vi "CheckValues.vi"(8 "error in (no error)":errorcluster, 11 "NHRDCPower in":refnum<class "NHRDCPower.lvclass">) -> (0 "error out":errorcluster, 3 "NHRDCPower out":refnum<class "NHRDCPower.lvclass">)   [LabVIEW 2018, in "AcPwrPlugins.lvlib" / "NHRDCPower.lvclass"]
uses:
  NHRDCPower.lvclass
  <vilib>/Utility/error.llb/Error Cluster From Error Code.vi
  <vilib>/ErrorRing/Error Ring.xnode
  <instrlib>/NHRDCPowerModule/NHRDCPowerModule/NHRDCPowerModule.lvlib
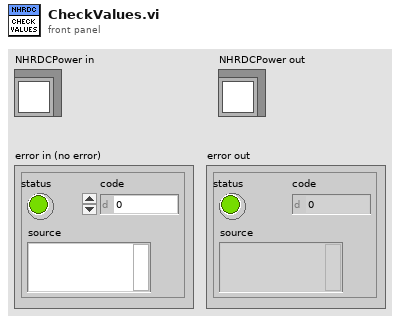
[diagram p1: front panel]
types:
  T1 = typedef "AcPwrPlugins.lvlib/NHRDCPower.lvclass/Device(s)Settings.ctl" = cluster{"Handle":string, "Name":string, "Phase Select":i32, "id query (Yes)":bool, "reset device (Yes)":bool, "Connected":bool, "Voltage Range (V)":dbl[], "Timing":cluster{"TimingOn":enum16{""}, "Hours":u32, "Minutes":u32, "Seconds":dbl, "CutoffVoltage":dbl}, "Simulate Instrument(T)":bool, "SlewRate":cluster{"Set Voltage Rate V/S":sgl, "Set Current Rate A/S":sgl, "Set Resistance Rate R/S":sgl, "Set Power Rate W/S":sgl}, "OutputSettings":cluster{"operating state (Off)":i32, "Voltage (V)":sgl, "Current (A)":sgl, "Resistance (Ohms)":sgl, "Power (W)":sgl, "Enable Voltage":bool, "Enable Current":bool, "Enable Resistance":bool, "Enable Power":bool, "Aperture Time (s)":sgl}, "Initial Battery Detect Voltage (0)":dbl, "SafetySettings":cluster{"SetWatchDog":bool, "Voltage (V)":sgl, "Current (A)":sgl, "Power (W)":sgl, "Voltage Delay (s)":sgl, "Current Delay (s)":sgl, "Power Delay (s)":sgl}}[]
  T2 = cluster{"Set Voltage Rate V/S":sgl, "Set Current Rate A/S":sgl, "Set Resistance Rate R/S":sgl, "Set Power Rate W/S":sgl}
  T3 = cluster{"operating state (Off)":i32, "Voltage (V)":sgl, "Current (A)":sgl, "Resistance (Ohms)":sgl, "Power (W)":sgl, "Enable Voltage":bool, "Enable Current":bool, "Enable Resistance":bool, "Enable Power":bool, "Aperture Time (s)":sgl}
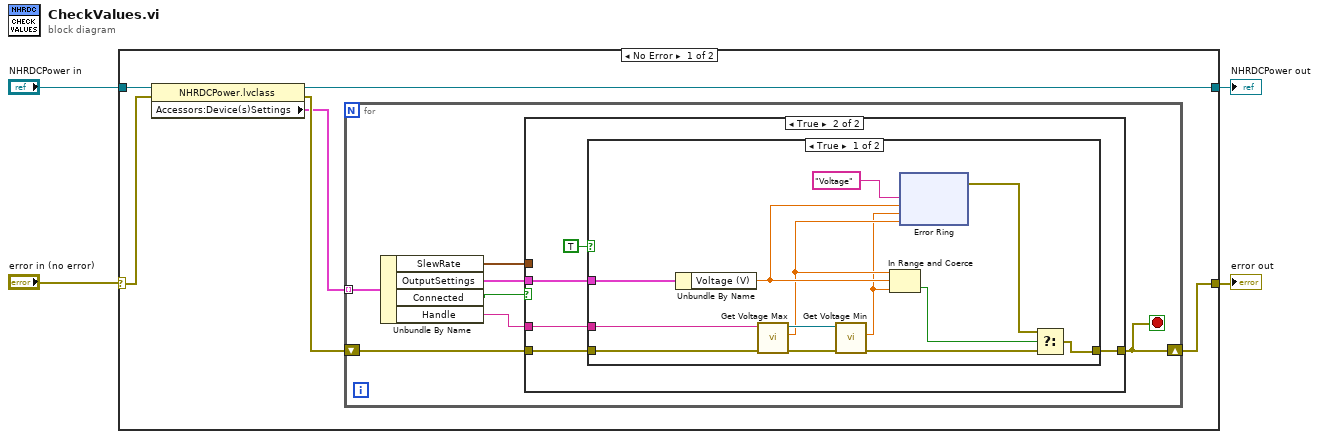
[diagram p0: block diagram]
diagram:
  n1 = case shown="No Error" "error in (no error)" {
    selector: "error in (no error)" -> [w9 w49]
    tunnel: [w8 w49] -> w1
    tunnel: [w10 w48] -> w3
    tunnel: "NHRDCPower in" -> [w6 w48]
    frame No Error {
      n2 = property class="NHRDCPower.lvclass"(reference=w6, error in=w9) -> (reference out=w10:refnum<class "NHRDCPower.lvclass">, error out=w7:errorcluster, "Accessors:Device(s)Settings"=w5:T1)
      n3 = for {
        tunnel: w5 -> [w17] mode=indexing
        shift-right: [w15] -> w8
        shift-left: w7 -> [w16]
        stop <- w15 stop-if-true
        n4 = Unbundle By Name(w17) -> ("SlewRate"=w11:T2, "OutputSettings"=w12:T3, "Connected"=w13:bool, "Handle"=w14:string)
        n5 = case shown="True" w13 {
          tunnel: w16 -> [w18 w23]
          tunnel: [w18 w20] -> w15
          tunnel: w14 -> [_ w22]
          tunnel: w12 -> [_ w21]
          tunnel: w11 -> [_ _]
          frame False {
          }
          frame True {
            n6 = case shown="True" TRUE {
              tunnel: w23 -> [w36 w47]
              tunnel: w22 -> [w35 _]
              tunnel: w21 -> [w32 _]
              tunnel: [w27 w47] -> w20
              frame True {
                n7 = Unbundle By Name(w32) -> ("Voltage (V)"=w31:sgl)
                n8 = call <instrlib>:"Get Voltage Max.vi"("error in (no error)"=w36, "instrument handle"=w35) -> ("error out"=w33:errorcluster, "maximum voltage"=w30:sgl, "instrument handle out"=w34:refnum<visa-resource-name>)  [unwired: 7 in]
                n9 = call <instrlib>:"Get Voltage Min.vi"("error in (no error)"=w33, "instrument handle"=w34) -> ("error out"=w28:errorcluster, "minimum voltage"=w29:sgl)  [unwired: 7 in, 1 out]
                n10 = In Range and Coerce(upper limit=w30, x=w31, lower limit=w29) -> (In Range?=w25:bool)  [unwired: 1 out]
                n11 = xnode "Error Ring"("parameter 0"="Voltage", "parameter 1"=w31, "parameter 2"=w29, "parameter 3"=w30) -> ("error out"=w26:errorcluster)
                n12 = Select(t=w26, s=w25, f=w28) -> (s? t:f=w27:errorcluster)
              }
              frame False {
              }
            }
          }
        }
      }
    }
    frame Error {
    }
  }
  "error out" <- w1
  "NHRDCPower out" <- w3
